vi "Dual_Fabry-Perot-tune-to.vi"() -> ()   [LabVIEW 2010]
panel:
  out "Temperature orders Et1":dbl[](array[numeric])=[30.0, 79.0289488656166, 110.46550450061054, 134.59725313809946, 155.53515021929462] format="%.2f"
  out "Temperature orders Et2":dbl[](array[numeric])=[30.0, 79.0289488656166, 110.46550450061054, 134.59725313809946, 155.53515021929462] format="%.2f"
  out "Order 1":dbl=30.25551322702913 format="%.1f"
  out "Order 2":dbl=30.25551322702913 format="%.1f"
  in  "Et1 T cur":dbl=83.2 format="%.2f"
  in  "Et2 T cur":dbl=101.0 format="%.2f"
  out "Set T Et2":dbl=90.0141317127521 format="%.2f"
  out "Set T Et 2":dbl=106.2543562252773 format="%.2f"
  in  "Wavelemgth":dbl=1.21 format="%#.2g"
  in  "Incrmt V1":dbl=50.0 format="%.2g"
  in  "Incrmt V2":dbl=50.0 format="%.2g"
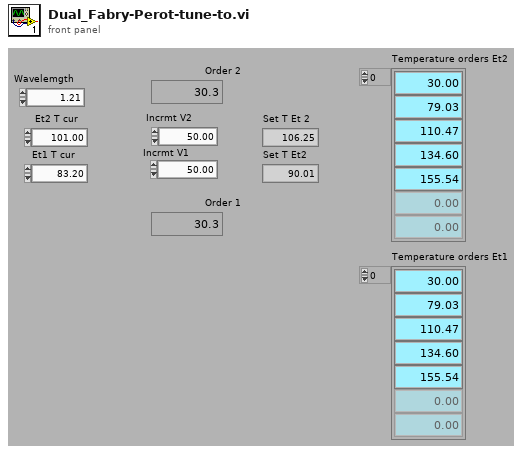
[diagram p1: front panel]
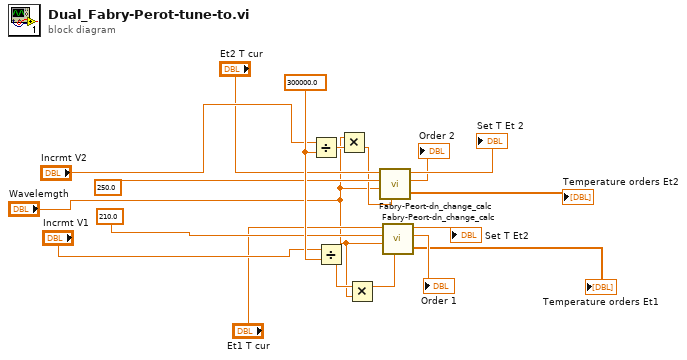
[diagram p0: block diagram]
diagram:
  w17 = 300000.0 ("Et thickness at 300K")
  n1 = Divide(x="Incrmt V2", y=w17) -> (x/y=w18:dbl)
  n2 = Divide(x="Incrmt V1", y=w17) -> (x/y=w10:dbl)
  n3 = Multiply(x="Wavelemgth", y=w18) -> (x*y=w7:dbl)
  n4 = Multiply(x=w10, y="Wavelemgth") -> (x*y=w6:dbl)
  n5 = call "Fabry-Peort-dn_change_calc.vi"("dLam chnage"=w7, "Wavelength"="Wavelemgth", "Et thickness at 300K"=250.0, "Et T(K)  initial"="Et2 T cur") -> ("Order"=→"Order 2":dbl, "Et T(K)  to"=→"Set T Et 2":dbl, "Temperature orders Et1 2"=→"Temperature orders Et2":dbl[])  [unwired: 3 in, 2 out]
  n6 = call "Fabry-Peort-dn_change_calc.vi"("dLam chnage"=w6, "Wavelength"="Wavelemgth", "Et thickness at 300K"=210.0, "Et T(K)  initial"="Et1 T cur") -> ("Order"=→"Order 1":dbl, "Et T(K)  to"=→"Set T Et2":dbl, "Temperature orders Et1 2"=→"Temperature orders Et1":dbl[])  [unwired: 3 in, 2 out]
